vi "Call sub.vi"() -> ()   [LabVIEW 2017]
uses:
  <vilib>/LVH/i3 JSON/i3-json.lvlib
panel:
  in  "JSON String":string="{\n  \"results\": [\n    {\n      \"statement_id\": 0,\n      \"series\": [\n        {\n          \"name\": \"databases\",\n          \"columns\": [\n            \"name\"\n          ],\n          \"values\": [\n            [\n              \"_internal\"\n            ],\n            [\n              \"labview\"\n            ]\n          ]\n        }\n      ]\n    }\n  ]\n}"
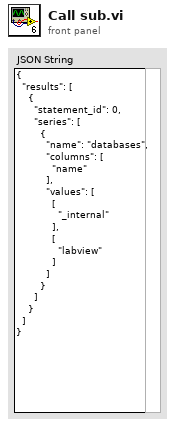
[diagram p1: front panel]
types:
  T1 = enum16{"open", "replace", "create", "open or create", "replace or create", "replace or create with confirmation"}
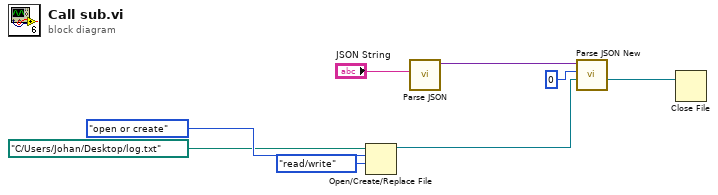
[diagram p0: block diagram]
diagram:
  n1 = Open/Create/Replace File(file path (use dialog)=path "C:/Users/Johan/Desktop/log.txt", operation (0:open)=T1."open or create", access (0:read/write)=enum16{"read/write", "read-only", "write-only"}."read/write") -> (refnum out=w4:refnum<file>)  [unwired: 3 in, 2 out]
  n2 = call <vilib>:"Parse JSON.vi"("JSON String"="JSON String") -> ("JSON Tree"=w7:variant)  [unwired: 7 in, 3 out]
  n3 = call "Parse JSON New.vi"("File ref in"=w4, "indent in"=0 ("indent in (0)"), "JSON Tree"=w7) -> ("File ref out"=w2:refnum<file>)  [unwired: 7 in, 1 out]
  n4 = Close File(refnum=w2) -> ()  [unwired: 1 in, 2 out]
